vi "ReadPort.vi"(8 "Error In":errorcluster, 11 "Kiethley 2602 In":refnum<visa-resource-name>) -> (0 "Error Out":errorcluster, 2 "Port":bool[](array[boolean]), 3 "Keithley 2602 Out":refnum<visa-resource-name>)   [LabVIEW 2012, in "Keithley-2602.lvlib"]
uses:
  Keithley-2602.lvlib
panel:
  out "number":dbl
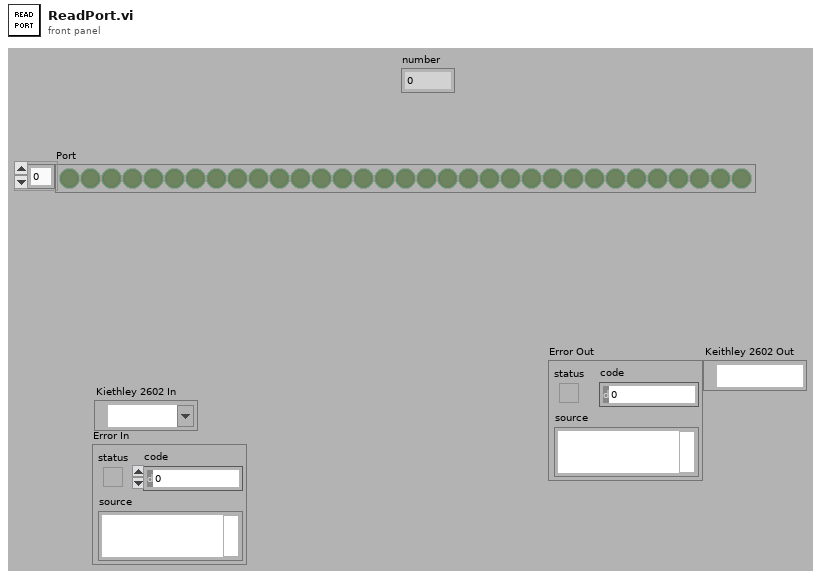
[diagram p1: front panel]
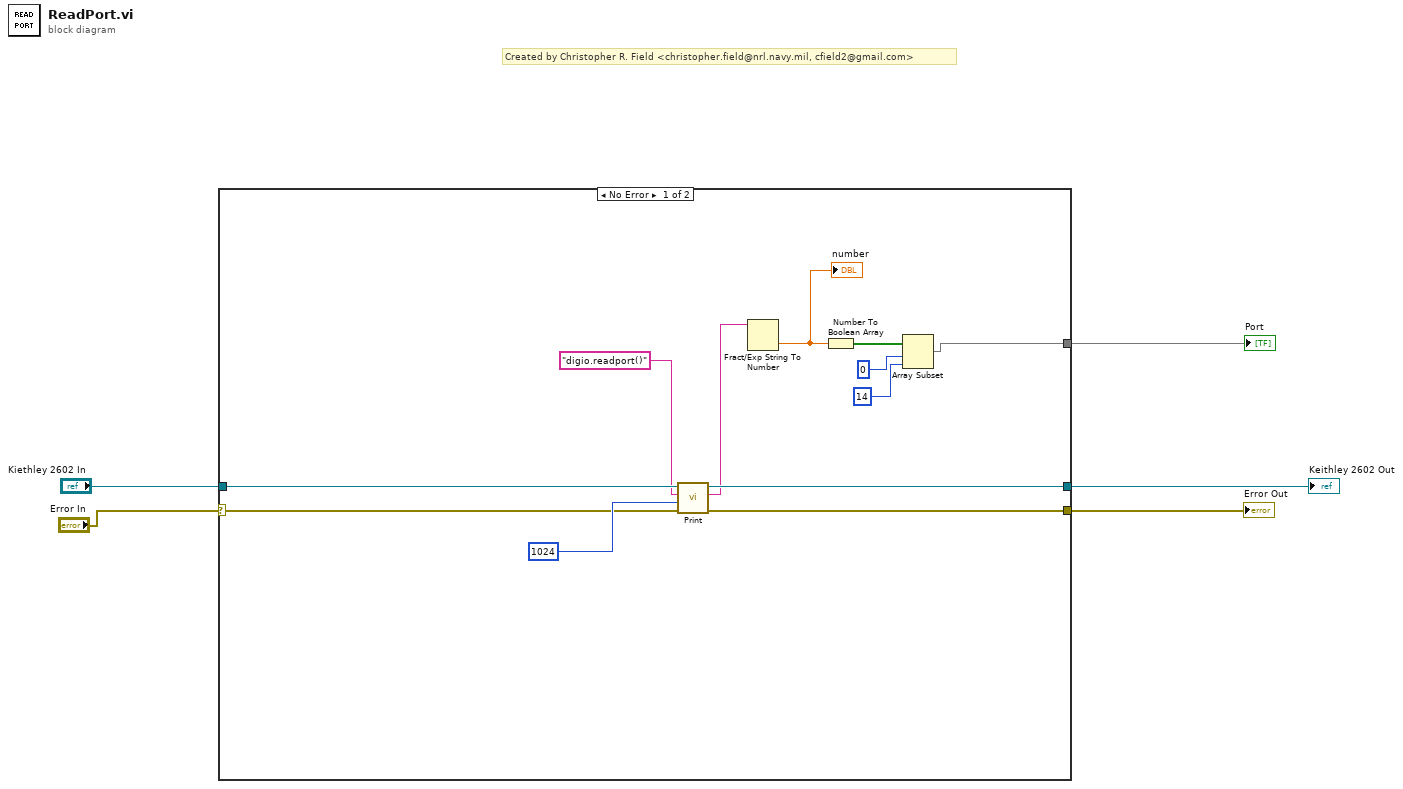
[diagram p0: block diagram]
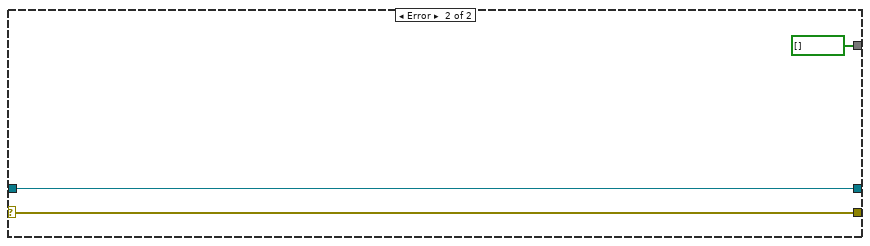
[diagram p2: hidden frame]
diagram:
  # "Created by Christopher R. Field <christopher.field@nrl.navy.mil, cfield2@gmail.com>"
  n1 = case shown="No Error" "Error In" {
    selector: "Error In" -> [w12 w18]
    tunnel: "Kiethley 2602 In" -> [w17 w19]
    tunnel: [w16 w19] -> w4
    tunnel: [w15 w18] -> w3
    tunnel: [w7 bool[] [] ("Boolean array")] -> w2
    frame No Error {
      n2 = call "Print.vi"("Error In"=w12, "Byte Count"=u32 1024, "Attribute"="digio.readport()", "Kiethley 2602 In"=w17) -> ("Error Out"=w15:errorcluster, "Output"=w11:string, "Keithley 2602 Out"=w16:refnum<visa-resource-name>)  [unwired: 5 in]
      n3 = Fract/Exp String To Number(string=w11) -> (number=w10:dbl)  [unwired: 3 in, 1 out]
      "number" <- w10
      n4 = Number To Boolean Array(number=w10) -> (Boolean array=w9:bool[])
      n5 = Array Subset(array=w9, index=0, length=14) -> (w7:bool[])
    }
    frame Error {
    }
  }
  "Error Out" <- w3
  "Keithley 2602 Out" <- w4
  "Port" <- w2
